vi "Signal2List.vi"(3 "nSignalIndex":u32, 5 "hMsg":u32) -> (0 "Value and Unit":string[](array[string]), 1 "Signal List":string[](array[string]))   [LabVIEW 2020]
uses:
  LVMessageHandle.vi
  bin/dbc_demo_api.dll
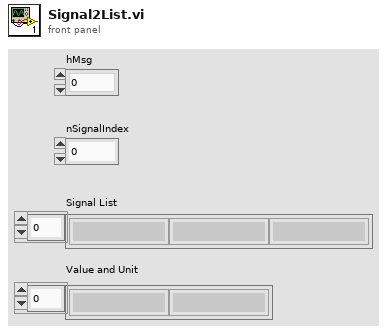
[diagram p1: front panel]
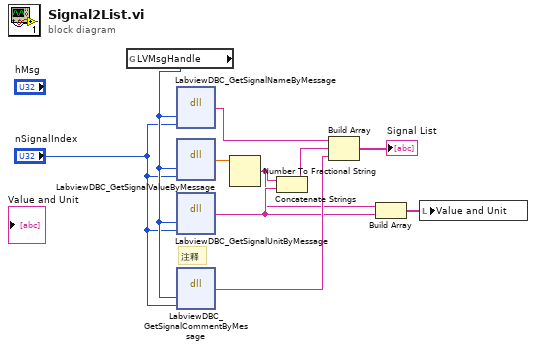
[diagram p0: block diagram]
diagram:
  # "注释"
  n1 = global read "LVMessageHandle.vi" "LVMsgHandle"() -> (w7:u32)
  n2 = dll-call lib="E:/Project/CANMaster/LabView/ZlgCan_Demo/bin/dbc_demo_api.dll" fn="LabviewDBC_GetSignalNameByMessage"("hMsg"=w7, "nSignalIndex"="nSignalIndex") -> ("strName"=w9:string)  [unwired: 5 in, 2 out]
  n3 = dll-call lib="E:/Project/CANMaster/LabView/ZlgCan_Demo/bin/dbc_demo_api.dll" fn="LabviewDBC_GetSignalValueByMessage"("hMsg"=w7, "nSignalIndex"="nSignalIndex") -> ("nValue"=w10:dbl)  [unwired: 5 in, 2 out]
  n4 = dll-call lib="E:/Project/CANMaster/LabView/ZlgCan_Demo/bin/dbc_demo_api.dll" fn="LabviewDBC_GetSignalUnitByMessage"("hMsg"=w7, "nSignalIndex"="nSignalIndex") -> ("strUnit"=w3:string)  [unwired: 5 in, 2 out]
  n5 = dll-call lib="E:/Project/CANMaster/LabView/ZlgCan_Demo/bin/dbc_demo_api.dll" fn="LabviewDBC_GetSignalCommentByMessage"("hMsg"=w7, "nSignalIndex"="nSignalIndex") -> ("strUnit"=w6:string)  [unwired: 5 in, 2 out]
  n6 = Number To Fractional String(number=w10) -> (F-format string=w2:string)  [unwired: 3 in]
  n7 = Concatenate Strings(w2, w3) -> (w8:string)
  n8 = Build Array(w9, w8, w6) -> (→"Signal List":string[])
  n9 = Build Array(w2, w3) -> (w1:string[])
  n10 = local write "Value and Unit"(w1) -> ()
